vi "forceTOdispl.vi"() -> ()   [LabVIEW 2011]
panel:
  out "Index":i32=2
  out "Thumb":i32=8
  out "Resultant Load Force":dbl
  out "Resultant Grip Force":dbl
  in  "force2displacemnt loop":bool
  out "subarray":dbl[][](array[numeric])=[[-0.0016047002615884648, 0.01962774474632563, 0.05388102532094477, -6.743846785846786e-05, 0.00032418926945717707, -0.0005535406771442331, 0.04658591023148378, 0.10359744995005873, 0.09177107845488962, 0.0007088752839781528, 0.0005091149263036229, -0.0001490476502194641, 0.038905158506793804, 0.041049406797413354, -0.2318981351133354, 0.0003706051814258798, 0.0003300945008706973, -0.0005507216127499452, 0.027342065946483203, 0.0063284743856839845, 0.011228207937424442, 0.0006610916509816831, 0.0007062586458297138, -0.00023219348927695451], [0.012798309188358076, 0.01092417773660311, 0.1272694001187903, -0.0001450092485733593, 0.0004738299906962181, -0.0007584704942989272, 0.012199878328640562, 0.0411633803945303, 0.03329774007675392, 0.0005124704259084759, 7.066848814634599e-05, 4.317642037141212e-05, 0.005299423293813158, -0.003370278256428499, -0.16521209929500077, 7.42094856124665e-05, 0.0005769248526913135, -0.0007510680850774225, 0.03254789740312213, 0.0032154344172637714, 0.06963187511481632, 0.00032399304516269787, -0.00019402019369577387, -0.0004224311720589758], [0.0017203445556565795, 0.023274075917015993, 0.039222554146342854, 5.02307106746716e-05, 5.724710676217142e-05, -0.0002546394943543632, 0.038336693856211336, 0.023469421725867298, 0.13860127402706493, 0.0014963025170351004, 0.0003243574753307975, -0.0003608981681178219, 0.027772762647286862, -0.038243515292141914, -0.13345045520840154, 9.913671599643043e-05, -0.0008372701697464751, -0.00023581040780558954, -0.01973027621419694, -0.022088178591826317, 0.02227800713172409, 0.0001368646707220728, 0.00013841632865222076, 0.00021519155444430486], [0.005408013485119663, 0.025269142586546195, -0.011506447727556098, -2.86214169226201e-05, 0.00016210482159179708, -0.0003062657735645173, -0.009895479653981737, 0.1206849398292366, 0.0745546395223249, 0.0010515350274939337, 0.0014625385879082678, -0.0001961015236909606, 0.016828393861908902, 0.009669503868452622, -0.050574579160010874, 7.920971038894653e-05, -0.0009941404806900968, -1.5702816965195018e-05, -0.021115457140616637, -0.016045240815307994, -0.029438026591823107, 0.0008189640530756826, 0.0007296784451514024, -1.5204687815181738e-05], [0.01115190770446399, 0.03670379676857504, 0.053987135563857425, 8.217673960425931e-05, 0.00019271400758203553, -0.0004781661136652485, 0.03326798457303174, 0.010491146668883025, -0.05122056548368485, 0.0007232903324966133, -0.0008570729392138996, 7.55099522331733e-05, -0.034266949639176605, -0.012241089683169651, -0.21451577126246754, 8.35103084577744e-05, 0.00021138857733046196, -0.0007826847508665894, -0.006804253322395364, 0.006594023866956576, 0.03333855024951253, 0.0009013987634261645, 0.00042766532098932196, 0.00011011269207797162], [0.019268240656181098, 0.030977709668134738, 0.030124780747790923, 2.1615041776338006e-05, 0.00040297862709188077, -0.0002877869957582795, 0.1074302009600285, 0.06742696695484761, 0.06413956229885383, 0.0019178257669685405, -0.0004284434387014629, -0.00013452364101756628, -0.027002371246654767, 0.009685154740743324, -0.05691670882486202, -0.00015283905251083568, 0.0007500746435299856, -0.00019091816134154659, 0.007730403501122321, 0.005287569848117169, 0.029276647486618575, 0.0007798916191205215, 0.00013216603713180397, -0.00034778124846752045], [0.011106503777328528, 0.022437646620986223, 0.06285462806248196, -4.220711725130722e-05, 0.0001071048785539649, -0.0003600837083180025, -0.03585624769568089, 0.10159239430406058, 0.033044137367145114, 0.0011445878617654408, 0.001456551067444766, -4.409777862374308e-06, -0.07814737243039128, 0.008376750644690014, 0.05992840508114507, -0.0006642828374729464, 0.000991671430226048, 0.00019742149066397614, 0.020635050521650898, -0.01908697049363589, -0.08002586349002709, 0.0007544280656719801, -8.343060734214193e-05, 2.672922988669045e-05], [0.004694513820669213, 0.019958593685490602, -0.05931338905984305, -0.00016146546080739402, 0.00031197690393288915, 0.00010907519352459618, -0.034291165830070365, -0.027944921695361093, -0.008038070133952954, 9.719711647102313e-05, -0.0010158802770549697, 0.00035354049540800667, -0.002764474884298997, 0.01715119342472284, 0.007148070321610785, 0.0003696295697706323, -0.0010631675337155033, -0.0011206366841255851, -0.018376332726581426, -0.009490108392591609, -0.022941526529401835, -0.00016996172094216696, 0.00021113347550948776, -0.0002058381676953041], [0.02152190723156776, -0.012475360554489745, 0.014317154725799858, -0.00012821723872848102, -0.00010144804083618626, -0.0002670509161738814, 0.08287674571699581, 0.1102199258674346, 0.18993600502125194, 0.0013232448341828752, 0.0006198024650922631, -0.0004810808835829848, -0.023481331116341198, 0.06279283487543294, -0.04140097663105311, 0.00010976198155341233, -0.0003293688251378183, -0.0009484470825381606, 0.0011932067018086917, -0.01345702513820748, 0.030125987341128455, -0.00011755926338180223, 0.0010380661254321998, -0.0002570805230206779], [0.013425963952264726, 0.030506283033742157, 0.1690182055294604, 0.0001222452324939653, 0.00040964377304742285, -0.0008257614692117129, -0.029320557955479238, 0.12389666757935941, 0.059181057992992725, 0.0005116848191208073, 0.0008266184837498157, -8.966850322436495e-06, 0.04203919634544276, 0.05420012053008159, 0.023064952003368756, 0.0005140855843844264, -0.0010773765414121492, -0.001108730990409999, -0.00821220027671831, -0.034998499190392836, -0.008470722665045245, -0.0004095754453320389, 0.0010658759922201459, 8.482416153973618e-05]]
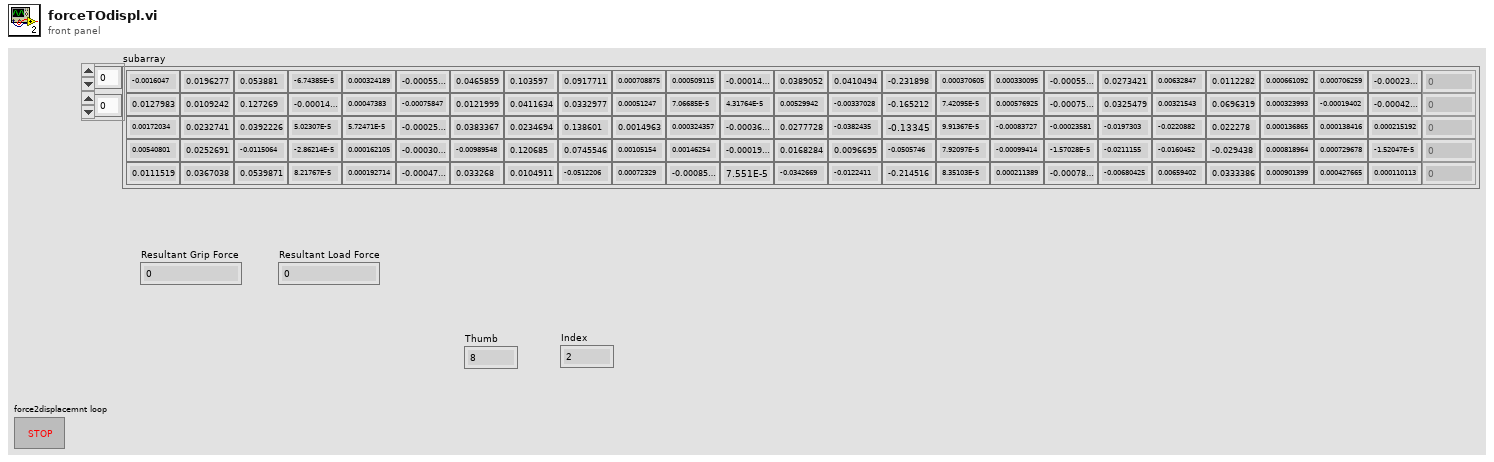
[diagram p1: front panel]
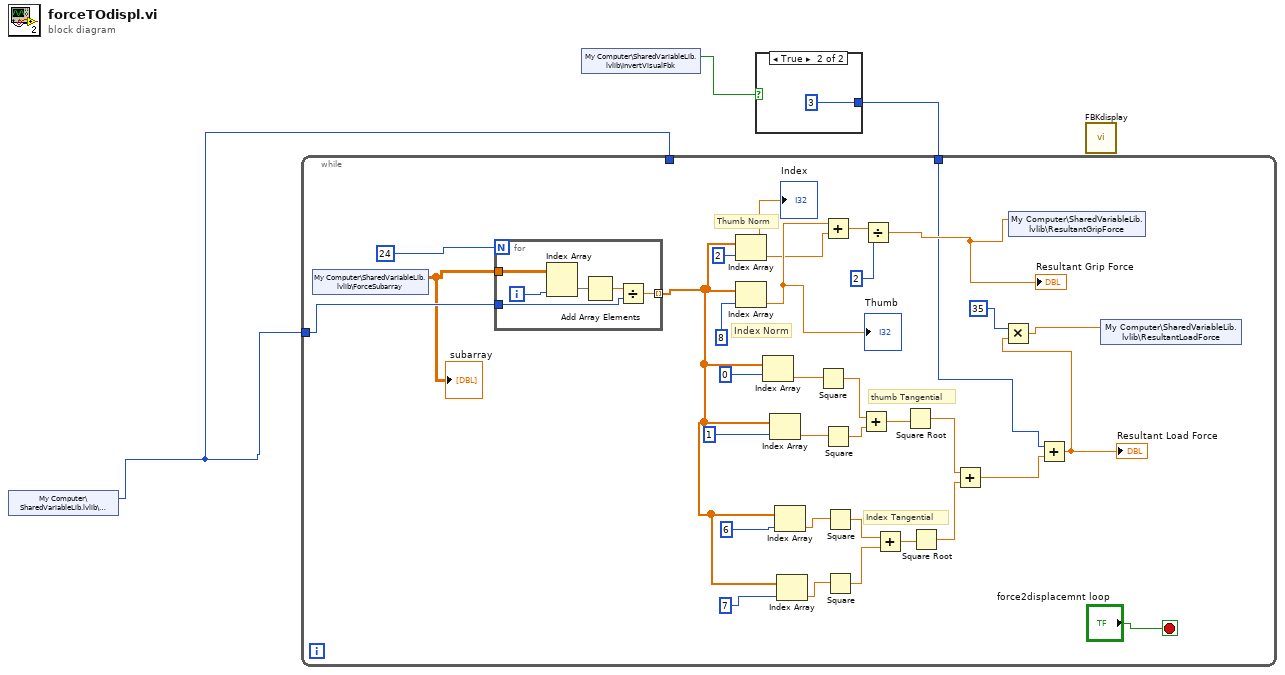
[diagram p0: block diagram]
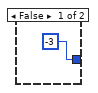
[diagram p2: hidden frame]
diagram:
  n1 = shared-variable "My Computer\\SharedVariableLib.lvlib\\Sample2Read"() -> (w3:i32)  [unwired: 1 in, 1 out]
  n2 = shared-variable "My Computer\\SharedVariableLib.lvlib\\InvertVisualFbk"() -> (w1:bool)  [unwired: 1 in, 1 out]
  n3 = case shown="True" w1 {
    tunnel: [-3 3] -> w2
    frame False {
    }
    frame True {
    }
  }
  n4 = while {
    tunnel: w3 -> [w37]
    tunnel: w3 -> [_]
    tunnel: w2 -> [w16]
    stop <- "force2displacemnt loop" stop-if-true
    # "Index Tangential"
    # "thumb Tangential"
    # "Index Norm"
    # "Thumb Norm"
    n5 = shared-variable "My Computer\\SharedVariableLib.lvlib\\ForceSubarray"() -> (w35:dbl[][])  [unwired: 1 in, 1 out]
    "subarray" <- w35
    n6 = for {
      N: 24 -> [_]
      tunnel: w35 -> [w43]
      tunnel: w37 -> [w42]
      tunnel: [w41] -> w26 mode=indexing
      i -> [w39]
      n7 = Index Array(array=w43, index (col)=w39) -> (element=w40:dbl[])  [unwired: 1 in]
      n8 = Add Array Elements(numeric array=w40) -> (sum=w44:dbl)
      n9 = Divide(x=w44, y=w42) -> (x/y=w41:dbl)
    }
    n10 = Index Array(array=w26, index=2) -> (element=w6:dbl)
    "Index" <- w6
    n11 = Index Array(array=w26, index=8) -> (element=w7:dbl)
    "Thumb" <- w7
    n12 = Index Array(array=w26, index=0) -> (element=w29:dbl)
    n13 = Index Array(array=w26, index=1) -> (element=w13:dbl)
    n14 = Index Array(array=w26, index=6) -> (element=w23:dbl)
    n15 = Index Array(array=w26, index=7) -> (element=w12:dbl)
    n16 = Square(x=w29) -> (x^2=w28:dbl)
    n17 = Add(x=w7, y=w6) -> (x+y=w32:dbl)
    n18 = Square(x=w13) -> (x^2=w14:dbl)
    n19 = Square(x=w23) -> (x^2=w22:dbl)
    n20 = Square(x=w12) -> (x^2=w21:dbl)
    n21 = Add(x=w28, y=w14) -> (x+y=w27:dbl)
    n22 = Divide(x=w32, y=2) -> (x/y=w17:dbl)
    "Resultant Grip Force" <- w17
    n23 = Add(x=w22, y=w21) -> (x+y=w20:dbl)
    n24 = Square Root(x=w27) -> (sqrt(x)=w10:dbl)
    n25 = Square Root(x=w20) -> (sqrt(x)=w9:dbl)
    n26 = Add(x=w10, y=w9) -> (x+y=w8:dbl)
    n27 = shared-variable "My Computer\\SharedVariableLib.lvlib\\ResultantGripForce"(w17) -> ()  [unwired: 1 in, 1 out]
    n28 = Add(x=w16, y=w8) -> (x+y=w15:dbl)
    "Resultant Load Force" <- w15
    n29 = Multiply(x=35, y=w15) -> (x*y=w19:dbl)
    n30 = shared-variable "My Computer\\SharedVariableLib.lvlib\\ResultantLoadForce"(w19) -> ()  [unwired: 1 in, 1 out]
  }
  n31 = call "FBKdisplay.vi"() -> ()  [unwired: 10 in]
